vi "Create Waveform Array.vi"(7 "channel info array":cluster{"Module":string, "Channel":string}[](array[cluster]) caption="通道信息数组", 8 "error in (no error)":errorcluster caption="错误输入（无错误）", 9 "samples to write":dbl[](array[numeric]) caption="待写入采样点", 10 "sampling period (s)":dbl caption="采样周期 (s)", 11 "Timestamp":timestamp caption="时间标识") -> (0 "error out":errorcluster caption="错误输出", 3 "Waveform Array":waveform(dbl)[](array[waveform]) caption="波形数据")   [LabVIEW 2015]
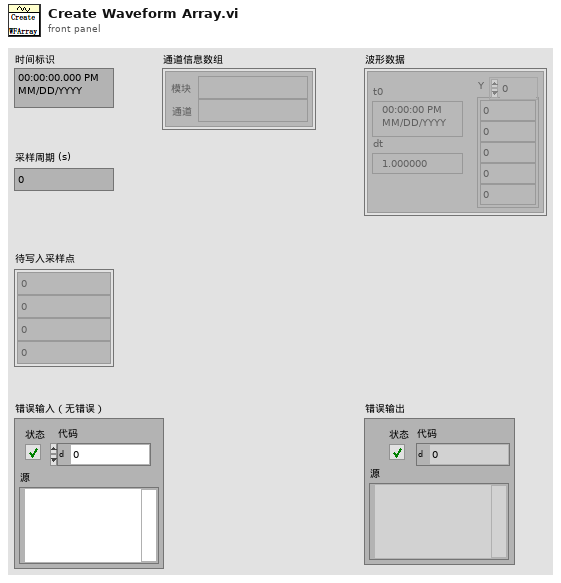
[diagram p1: front panel]
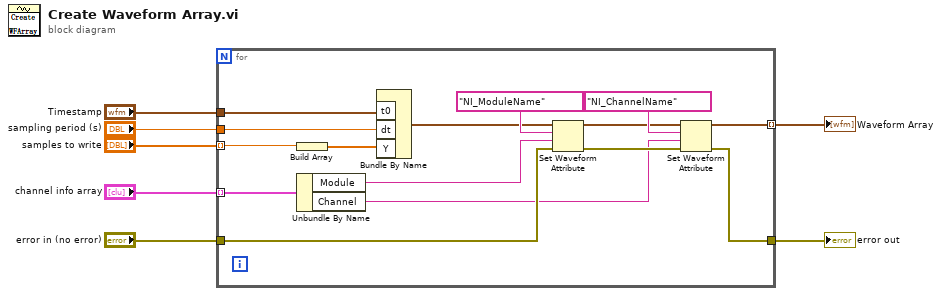
[diagram p0: block diagram]
diagram:
  n1 = for {
    tunnel: [w22] -> w3 mode=indexing
    tunnel: "error in (no error)" -> [w21]
    tunnel: [w19] -> w6
    tunnel: "samples to write" -> [w14] mode=indexing
    tunnel: "Timestamp" -> [w13]
    tunnel: "channel info array" -> [w12] mode=indexing
    tunnel: "sampling period (s)" -> [w8]
    n2 = Build Array(w14) -> (w9:dbl[])
    n3 = Unbundle By Name(w12) -> ("Module"=w10:string, "Channel"=w11:string)
    n4 = Bundle By Name("t0"=w13, "dt"=w8, "Y"=w9) -> (w16:waveform(dbl))  [unwired: 1 in]
    n5 = Set Waveform Attribute(4:w21, 5:w10, 6:"NI_ModuleName", 7:w16) -> (0:w20:errorcluster, 3:w15:waveform(dbl))  [unwired: 1 out]
    n6 = Set Waveform Attribute(4:w20, 5:w11, 6:"NI_ChannelName", 7:w15) -> (0:w19:errorcluster, 3:w22:waveform(dbl))  [unwired: 1 out]
  }
  "error out" <- w6
  "Waveform Array" <- w3
